vi "加标模块单控对话框.vi"(11 "标题":string="加标模块") -> ()   [LabVIEW 2016, in "质控单元.lvlib"]
panel:
  out "流程":enum16{"润洗", "进样", "加标", "搅拌", "排液"}(ring)
  in  "加标":bool
  in  "排液":bool
  in  "搅拌":bool
  in  "进样":bool
  in  "润洗":bool
  in  "慢速到液位":bool
  in  "排液":bool
  in  "退出":bool
  in  "柱塞泵":bool
  in  "排液":bool
  in  "搅拌":bool
  in  "进样调速":bool
  in  "进样":bool
  in  "停止":bool
  in  "加标启动":bool
  # "单步控制"
  # "流程步骤"
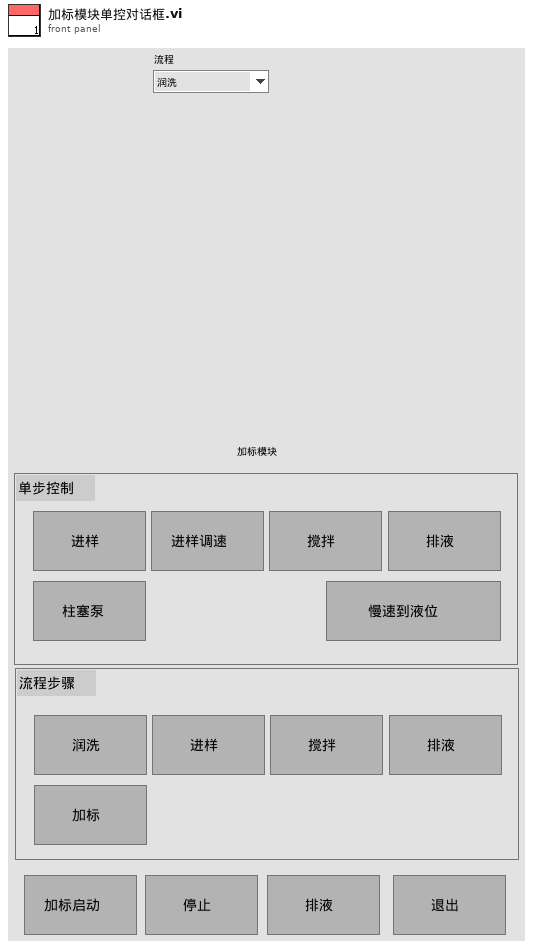
[diagram p1: front panel]
types:
  T1 = cluster{"氨氮":u8, "总磷":u8, "总氮":u8, "CODMn":u8, "CODCr":u8}
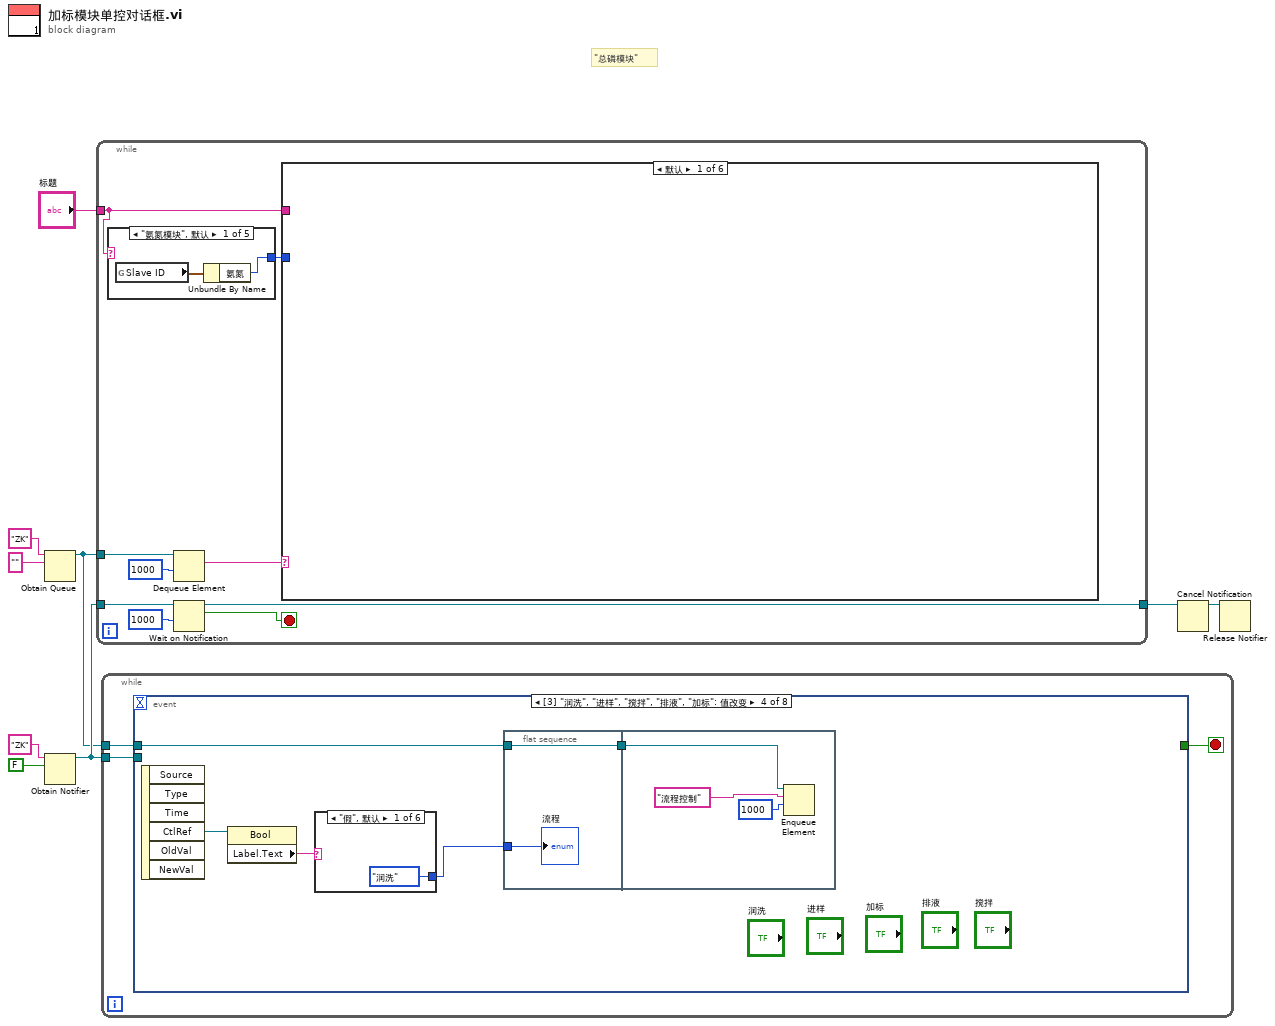
[diagram p0: block diagram]
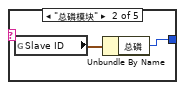
[diagram p2: hidden frame]
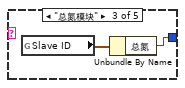
[diagram p3: hidden frame]
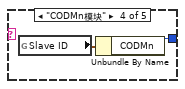
[diagram p4: hidden frame]
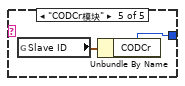
[diagram p5: hidden frame]
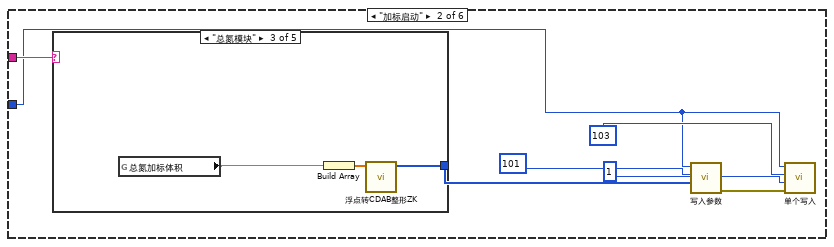
[diagram p6: hidden frame]
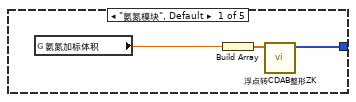
[diagram p7: hidden frame]
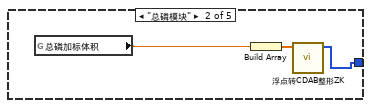
[diagram p8: hidden frame]
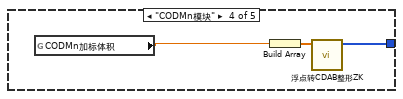
[diagram p9: hidden frame]
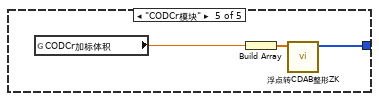
[diagram p10: hidden frame]
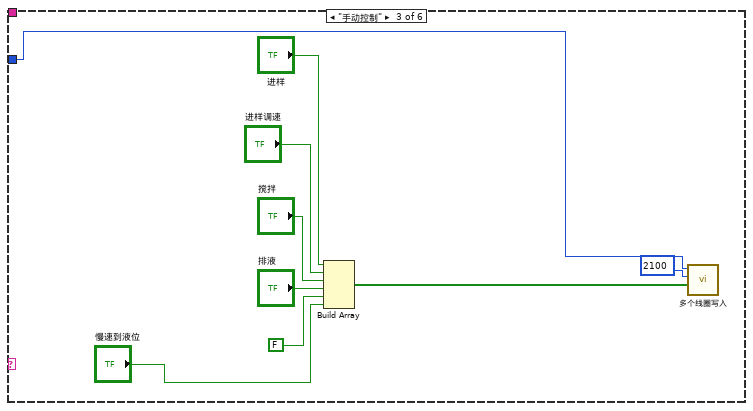
[diagram p11: hidden frame]
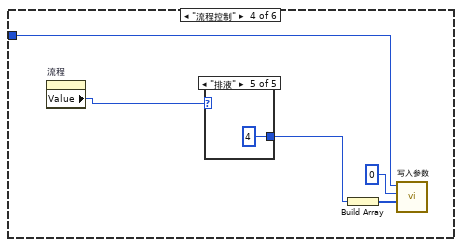
[diagram p12: hidden frame]
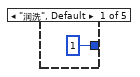
[diagram p13: hidden frame]
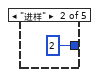
[diagram p14: hidden frame]
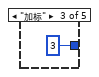
[diagram p15: hidden frame]
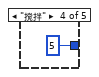
[diagram p16: hidden frame]
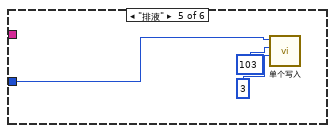
[diagram p17: hidden frame]
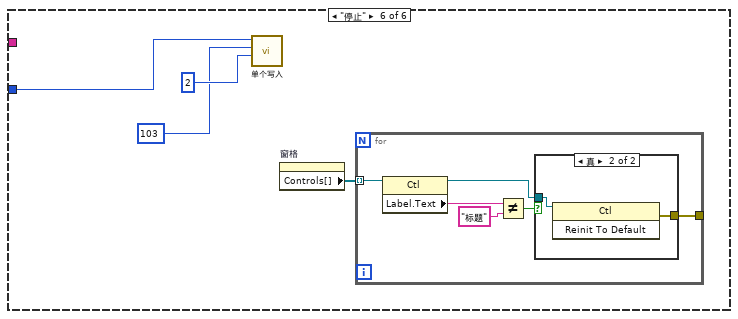
[diagram p18: hidden frame]
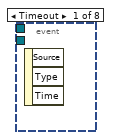
[diagram p20: hidden frame]
diagram:
  # "\"总磷模块\""
  n1 = Obtain Queue(name (unnamed)="ZK" ("名称（未命名）"), element data type="" ("名称（未命名）")) -> (queue out=w2:refnum<queue>)  [unwired: 3 in, 2 out]
  n2 = Obtain Notifier(name (unnamed)="ZK" ("名称（未命名）"), notification data type=FALSE) -> (notifier out=w7:refnum<notifier>)  [unwired: 2 in, 2 out]
  n3 = while {
    tunnel: w7 -> [w18]
    tunnel: [w16] -> w6
    tunnel: w2 -> [w15]
    tunnel: "标题" -> [w11]
    stop <- w17 stop-if-true
    n4 = case shown="\"氨氮模块\", 默认" w11 {
      tunnel: [w19 w21 w23 w25 w27] -> w10
      frame "氨氮模块", Default {
        n5 = global read "断电保存全局.vi" "Slave ID"() -> (w20:T1)
        n6 = Unbundle By Name(w20) -> ("氨氮"=w19:u8)
      }
      frame "总磷模块" {
        n7 = global read "断电保存全局.vi" "Slave ID"() -> (w22:T1)
        n8 = Unbundle By Name(w22) -> ("总磷"=w21:u8)
      }
      frame "总氮模块" {
        n9 = global read "断电保存全局.vi" "Slave ID"() -> (w24:T1)
        n10 = Unbundle By Name(w24) -> ("总氮"=w23:u8)
      }
      frame "CODMn模块" {
        n11 = global read "断电保存全局.vi" "Slave ID"() -> (w26:T1)
        n12 = Unbundle By Name(w26) -> ("CODMn"=w25:u8)
      }
      frame "CODCr模块" {
        n13 = global read "断电保存全局.vi" "Slave ID"() -> (w28:T1)
        n14 = Unbundle By Name(w28) -> ("CODCr"=w27:u8)
      }
    }
    n15 = Dequeue Element(queue=w15, timeout in ms (-1)=1000 ("超时毫秒(-1)")) -> (element=w14:string)  [unwired: 1 in, 3 out]
    n16 = Wait on Notification(notifier=w18, timeout in ms (-1)=1000 ("超时毫秒(-1)")) -> (notifier out=w16:refnum<notifier>, notification=w17:bool)  [unwired: 2 in, 2 out]
    n17 = case shown="默认" w14 {
      tunnel: w11 -> [_ w30 _ _ _ _]
      tunnel: w10 -> [_ w29 w51 w61 w70 w73]
      frame Default {
      }
      frame "加标启动" {
        n18 = case shown="\"总氮模块\"" w30 {
          tunnel: [w37 w41 w43 w46 w49] -> w32
          frame "氨氮模块", Default {
            n19 = global read "加标回收状态全局变量.vi" "氨氮加标体积"() -> (w36:dbl)
            n20 = Build Array(w36) -> (w38:dbl[])
            n21 = call "浮点转CDAB整形ZK.vi"("浮点数"=w38) -> ("CDAB整形输出"=w37:u16[])  [unwired: 10 in]
          }
          frame "总磷模块" {
            n22 = global read "加标回收状态全局变量.vi" "总磷加标体积"() -> (w39:dbl)
            n23 = Build Array(w39) -> (w40:dbl[])
            n24 = call "浮点转CDAB整形ZK.vi"("浮点数"=w40) -> ("CDAB整形输出"=w41:u16[])  [unwired: 10 in]
          }
          frame "总氮模块" {
            n25 = global read "加标回收状态全局变量.vi" "总氮加标体积"() -> (w42:dbl)
            n26 = Build Array(w42) -> (w44:dbl[])
            n27 = call "浮点转CDAB整形ZK.vi"("浮点数"=w44) -> ("CDAB整形输出"=w43:u16[])  [unwired: 10 in]
          }
          frame "CODMn模块" {
            n28 = global read "加标回收状态全局变量.vi" "CODMn加标体积"() -> (w45:dbl)
            n29 = Build Array(w45) -> (w47:dbl[])
            n30 = call "浮点转CDAB整形ZK.vi"("浮点数"=w47) -> ("CDAB整形输出"=w46:u16[])  [unwired: 10 in]
          }
          frame "CODCr模块" {
            n31 = global read "加标回收状态全局变量.vi" "CODCr加标体积"() -> (w48:dbl)
            n32 = Build Array(w48) -> (w50:dbl[])
            n33 = call "浮点转CDAB整形ZK.vi"("浮点数"=w50) -> ("CDAB整形输出"=w49:u16[])  [unwired: 10 in]
          }
        }
        n34 = call "写入参数.vi"("values"=w32, "starting address"=u16 101, "Slave ID"=w29) -> ("error out"=w31:errorcluster)  [unwired: 8 in]
        n35 = call "单个写入.vi"("Error in"=w31, "value"=u16 1, "address"=u16 103, "Slave ID"=w29) -> ()  [unwired: 7 in, 1 out]
      }
      frame "手动控制" {
        n36 = Build Array("进样", "进样调速", "搅拌", "排液", FALSE ("元素"), "慢速到液位") -> (w57:bool[])
        n37 = call "多个线圈写入.vi"("values"=w57, "starting address"=u16 2100, "Slave ID"=w51) -> ()  [unwired: 8 in, 1 out]
      }
      frame "流程控制" {
        n38 = property on="流程" class="Enum (严格)"() -> ("Value"=w60:enum16{"润洗", "进样", "加标", "搅拌", "排液"})  [unwired: 2 in, 2 out]
        n39 = case shown="\"排液\"" w60 {
          tunnel: [u16 1 ("quantity") u16 2 ("quantity") u16 3 ("quantity") u16 5 ("quantity") u16 4 ("quantity")] -> w63
          frame "润洗", Default {
          }
          frame "进样" {
          }
          frame "加标" {
          }
          frame "搅拌" {
          }
          frame "排液" {
          }
        }
        n40 = Build Array(w63) -> (w62:u16[])
        n41 = call "写入参数.vi"("values"=w62, "starting address"=u16 0, "Slave ID"=w61) -> ()  [unwired: 8 in, 1 out]
      }
      frame "排液" {
        n42 = call "单个写入.vi"("value"=u16 3, "address"=u16 103, "Slave ID"=w70) -> ()  [unwired: 8 in, 1 out]
      }
      frame "停止" {
        n43 = call "单个写入.vi"("value"=u16 2, "address"=u16 103, "Slave ID"=w73) -> ()  [unwired: 8 in, 1 out]
        n44 = property on="窗格" class="Pane"() -> ("Controls[]"=w74:refnum<vi>[])  [unwired: 2 in, 2 out]
        n45 = for {
          tunnel: w74 -> [w81] mode=indexing
          tunnel: [w82] -> _
          n46 = property class="Ctl"(reference=w81) -> (reference out=w77:refnum<vi>, "Label.Text"=w80:string)  [unwired: 1 in, 1 out]
          n47 = Not Equal?(x=w80, y="标题") -> (x != y?=w78:bool)
          n48 = case shown="真" w78 {
            tunnel: [_ w84] -> w82
            tunnel: w77 -> [_ w83]
            frame False {
            }
            frame True {
              n49 = invoke class="Ctl" method="Reinit To Default"(reference=w83) -> (error out=w84:errorcluster)  [unwired: 2 in, 2 out]
            }
          }
        }
      }
    }
  }
  n50 = while {
    tunnel: w7 -> [w86]
    tunnel: w2 -> [w85]
    stop <- w87 stop-if-true
    n51 = event shown="[3] \"润洗\", \"进样\", \"搅拌\", \"排液\", \"加标\": 值改变" {
      selector: _ -> [_ _ _ _ _ _ _ _]
      dyn-events: _ -> [_ _ _ _ _ _ _ _]
      timeout: _ -> [_ _ _ _ _ _ _ _]
      tunnel: [_ _ _ _ _ _ _ TRUE] -> w87
      tunnel: w86 -> [_ _ _ _ _ _ _ w119]
      tunnel: w85 -> [_ w90 w91 w98 _ w110 w115 w118]
      event Timeout {
        n52 = event-data() -> ()  [unwired: 1 in, 3 out]
      }
      event "加标启动": Value Change {
        n53 = event-data() -> ()  [unwired: 1 in, 4 out]
        n54 = Enqueue Element(queue=w90, element="加标启动" ("元素"), timeout in ms (-1)=1000 ("超时毫秒(-1)")) -> ()  [unwired: 1 in, 3 out]
      }
      event "进样", "进样调速", "搅拌", "排液", "慢速到液位": Value Change {
        n55 = event-data() -> ()  [unwired: 1 in, 5 out]
        n56 = Enqueue Element(queue=w91, element="手动控制" ("元素"), timeout in ms (-1)=1000 ("超时毫秒(-1)")) -> ()  [unwired: 1 in, 3 out]
      }
      event "润洗", "进样", "搅拌", "排液", "加标": Value Change {
        n57 = event-data() -> ("CtlRef"=w97:refnum<vi>)  [unwired: 1 in, 5 out]
        n58 = property class="Bool"(reference=w97) -> ("Label.Text"=w96:string)  [unwired: 1 in, 2 out]
        n59 = case shown="\"假\", 默认" w96 {
          tunnel: [enum16{"润洗", "进样", "加标", "搅拌", "排液"}."润洗" ("流程") enum16{"润洗", "进样", "加标", "搅拌", "排液"}."润洗" ("流程") enum16{"润洗", "进样", "加标", "搅拌", "排液"}."进样" ("流程") enum16{"润洗", "进样", "加标", "搅拌", "排液"}."搅拌" ("流程") enum16{"润洗", "进样", "加标", "搅拌", "排液"}."排液" ("流程") enum16{"润洗", "进样", "加标", "搅拌", "排液"}."加标" ("流程")] -> w94
          frame "假", Default {
          }
          frame "润洗" {
          }
          frame "进样" {
          }
          frame "搅拌" {
          }
          frame "排液" {
          }
          frame "加标" {
          }
        }
        n60 = flat-sequence {
          tunnel: w98 -> [w100]
          tunnel: [w100] -> w95
          tunnel: w94 -> [w99]
          tunnel: w95 -> [w102]
          frame #0 {
            "流程" <- w99
          }
          frame #1 {
            n61 = Enqueue Element(queue=w102, element="流程控制" ("元素"), timeout in ms (-1)=1000 ("超时毫秒(-1)")) -> ()  [unwired: 1 in, 3 out]
          }
        }
      }
      event "柱塞泵": Value Change {
        n62 = event-data() -> ()  [unwired: 1 in, 6 out]
        n63 = call "柱塞泵调试界面.vi"() -> ()  [unwired: 16 in]
      }
      event "排液": Value Change {
        n64 = event-data() -> ()  [unwired: 1 in, 6 out]
        n65 = Enqueue Element(queue=w110, element="排液" ("元素"), timeout in ms (-1)=1000 ("超时毫秒(-1)")) -> ()  [unwired: 1 in, 3 out]
      }
      event "停止": Value Change {
        n66 = event-data() -> ()  [unwired: 1 in, 5 out]
        n67 = Flush Queue(queue=w115) -> (queue out=w114:refnum<queue>)  [unwired: 1 in, 2 out]
        n68 = Enqueue Element(queue=w114, element="停止" ("元素"), timeout in ms (-1)=1000 ("超时毫秒(-1)")) -> ()  [unwired: 1 in, 3 out]
      }
      event "退出": Value Change; Panel Close {
        n69 = event-data() -> ()  [unwired: 1 in, 3 out]
        n70 = Send Notification(notification=TRUE ("通知"), notifier=w119) -> ()  [unwired: 1 in, 2 out]
        n71 = Flush Queue(queue=w118) -> (queue out=w117:refnum<queue>)  [unwired: 1 in, 2 out]
        n72 = Two Button Dialog(message="请确认是否退出，退出仪器将停止运行" ("消息"), 1:"N" ("F按钮名称（“取消”）"), 2:"Y" ("T按钮名称（“确定”）")) -> (T button?=w121:bool)
        n73 = case shown="真" w121 {
          tunnel: w117 -> [_ w126]
          frame False {
          }
          frame True {
            n74 = Enqueue Element(queue=w126, element="停止" ("元素"), timeout in ms (-1)=1000 ("超时毫秒(-1)")) -> ()  [unwired: 1 in, 3 out]
          }
        }
      }
    }
  }
  n75 = Cancel Notification(0:w6) -> (8:w5:refnum<notifier>)  [unwired: 1 in, 2 out]
  n76 = Release Notifier(notifier=w5) -> ()  [unwired: 2 in, 3 out]
